vi "Open_Windows_File.vi"(0 "selected path":path) -> ()   [LabVIEW 2011]
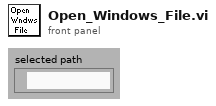
[diagram p1: front panel]
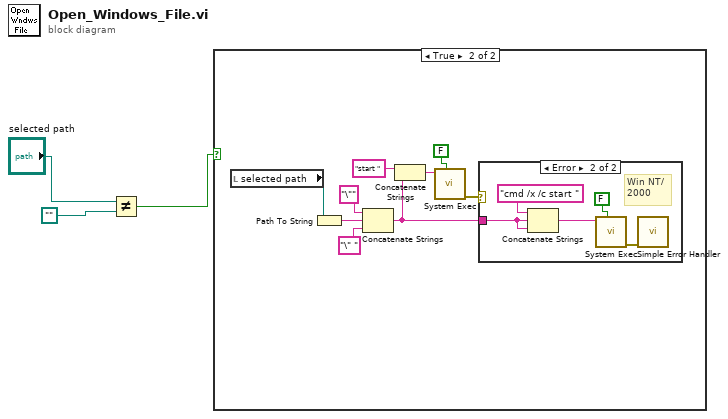
[diagram p0: block diagram]
diagram:
  n1 = Not Equal?(x="selected path", y=path "") -> (x != y?=w2:bool)
  n2 = case shown="True" w2 {
    frame False {
    }
    frame True {
      n3 = local read "selected path"() -> (w4:path)
      n4 = Path To String(path=w4) -> (string=w5:string)
      n5 = Concatenate Strings("\"" ("Substring"), w5, "\" " ("Substring")) -> (w7:string)
      n6 = Concatenate Strings("start " ("Substring"), w7) -> (w8:string)
      n7 = call <vilib>:"System Exec.vi"("wait until completion? (T)"=FALSE ("Wait until done"), "command line"=w8) -> ("error out"=w9:errorcluster)  [unwired: 6 in, 3 out]
      n8 = case shown="Error" w9 {
        tunnel: w7 -> [_ w13]
        frame No Error {
          # "Win 95/98/Me"
        }
        frame Error {
          # "Win NT/\n2000"
          n9 = Concatenate Strings("cmd /x /c start ", w13, w13) -> (w15:string)
          n10 = call <vilib>:"System Exec.vi"("wait until completion? (T)"=FALSE ("Wait until done"), "command line"=w15) -> ("error out"=w14:errorcluster)  [unwired: 6 in, 3 out]
          n11 = call <vilib>:"Simple Error Handler.vi"("error in (no error)"=w14) -> ()  [unwired: 4 in, 5 out]
        }
      }
    }
  }
